vi "Add Tag.vi"() -> ()   [LabVIEW 2017, in "Mustache.lvlib" / "Parser.lvclass"]
uses:
  Parser.lvclass
  Public/Controls/Token Types.ctl
panel:
  out "Parser Out":refnum<class "Parser.lvclass">
  out "Error Out":errorcluster
  in  "Error In":errorcluster
  in  "Parser In":refnum<class "Parser.lvclass">
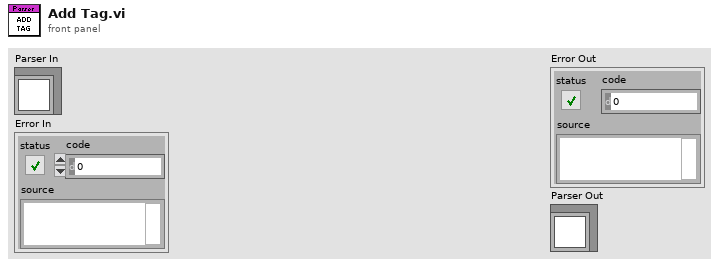
[diagram p1: front panel]
types:
  T1 = typedef "Mustache.lvlib/Parser.lvclass/Token Types.ctl" = enum16{"Text", "Escaped Tag", "Unescaped Tag", "Section", "Incomplete Section", "Partial"}
  T2 = typedef "Mustache.lvlib/Parser.lvclass/Token.ctl" = cluster{"Type":T1, "Data":variant}
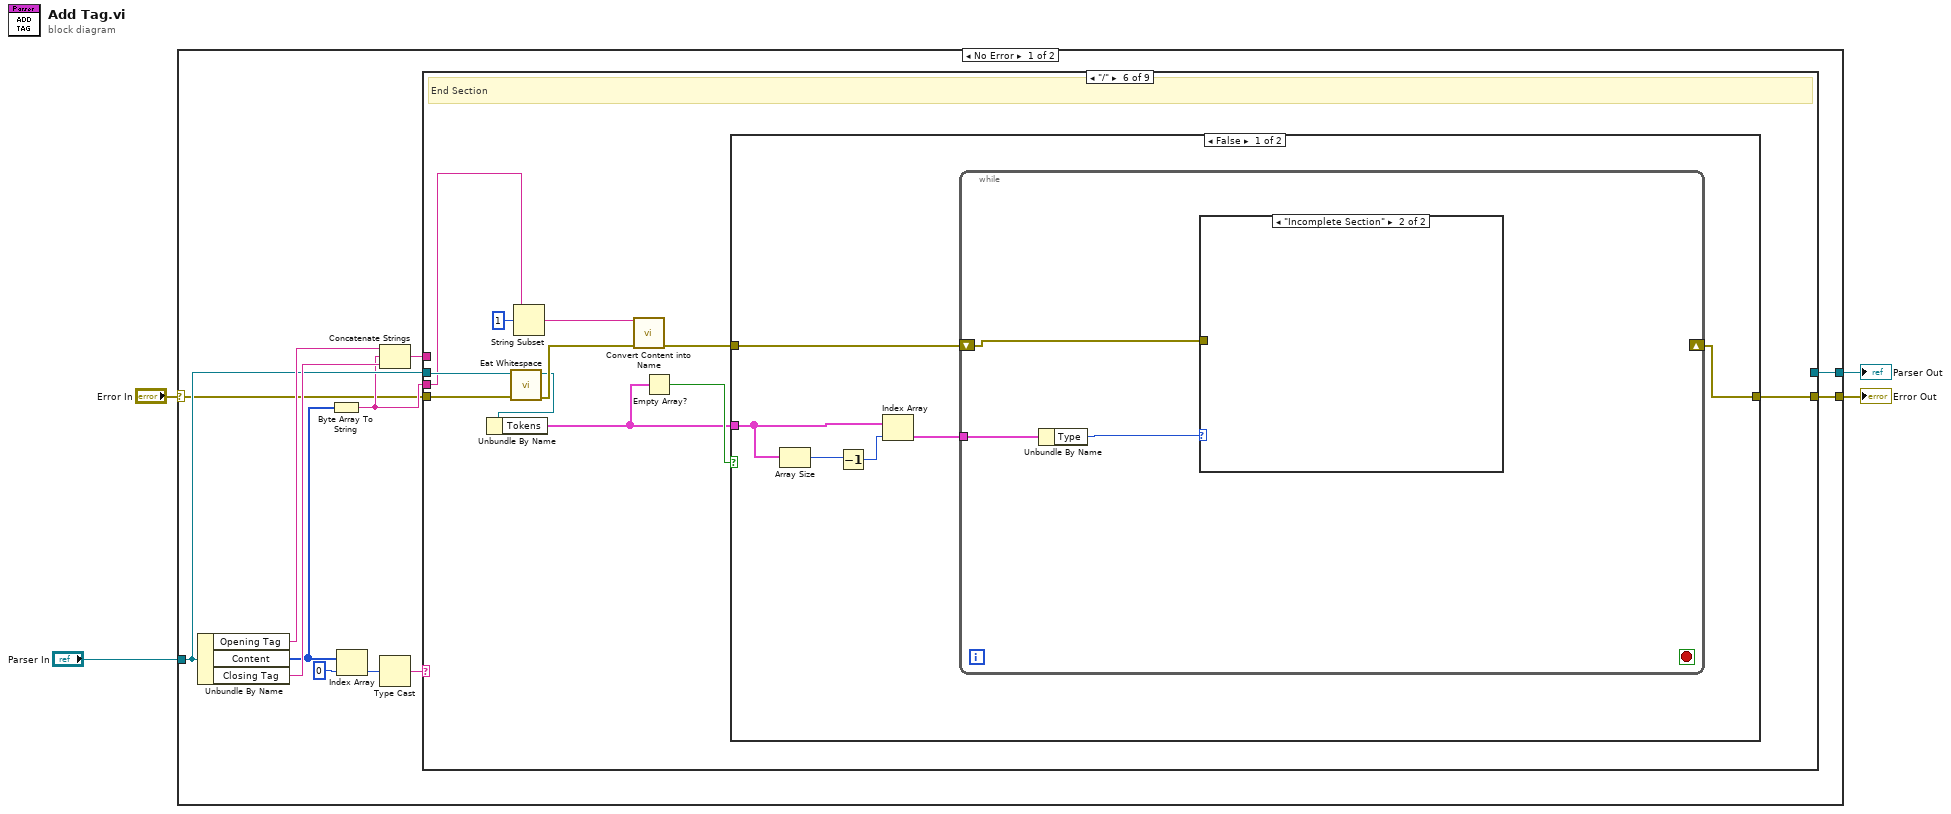
[diagram p0: block diagram]
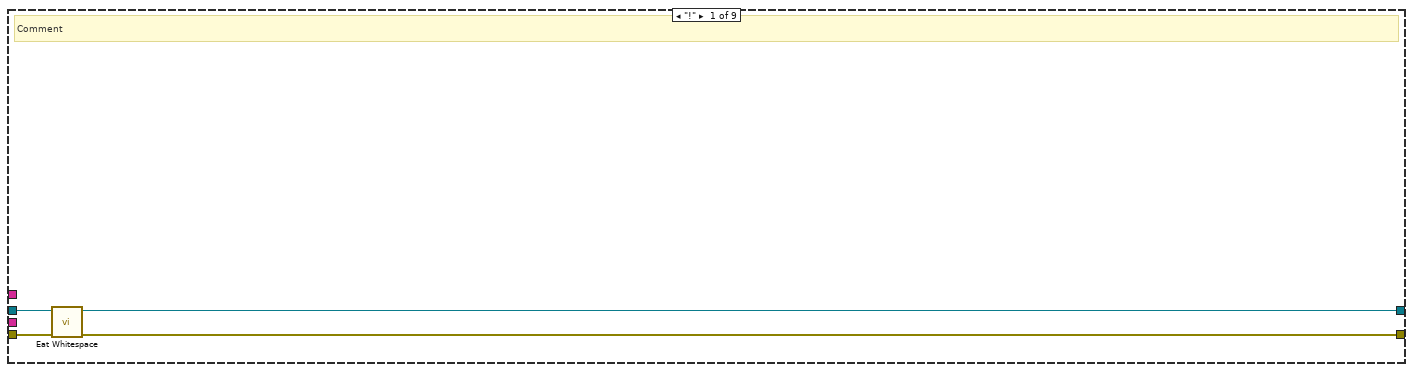
[diagram p2: hidden frame]
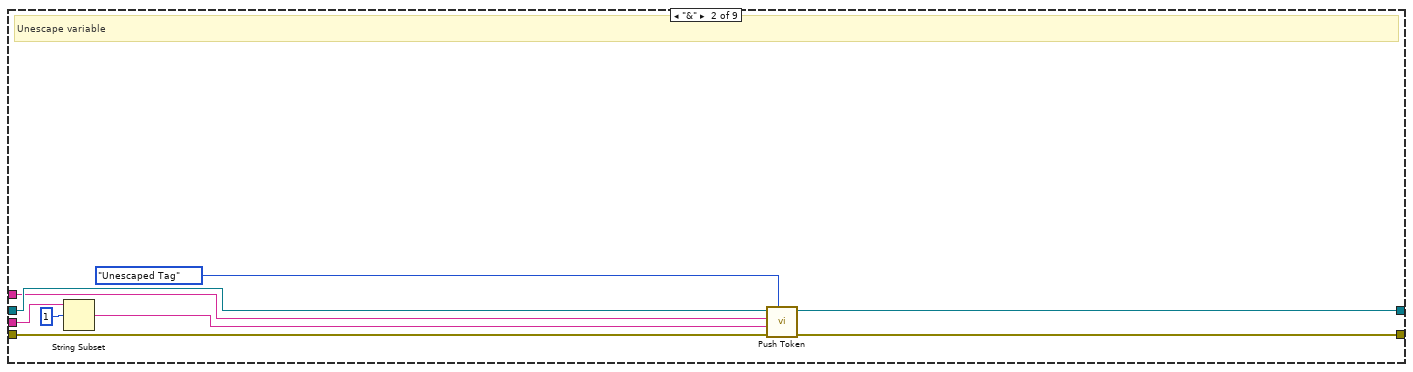
[diagram p3: hidden frame]
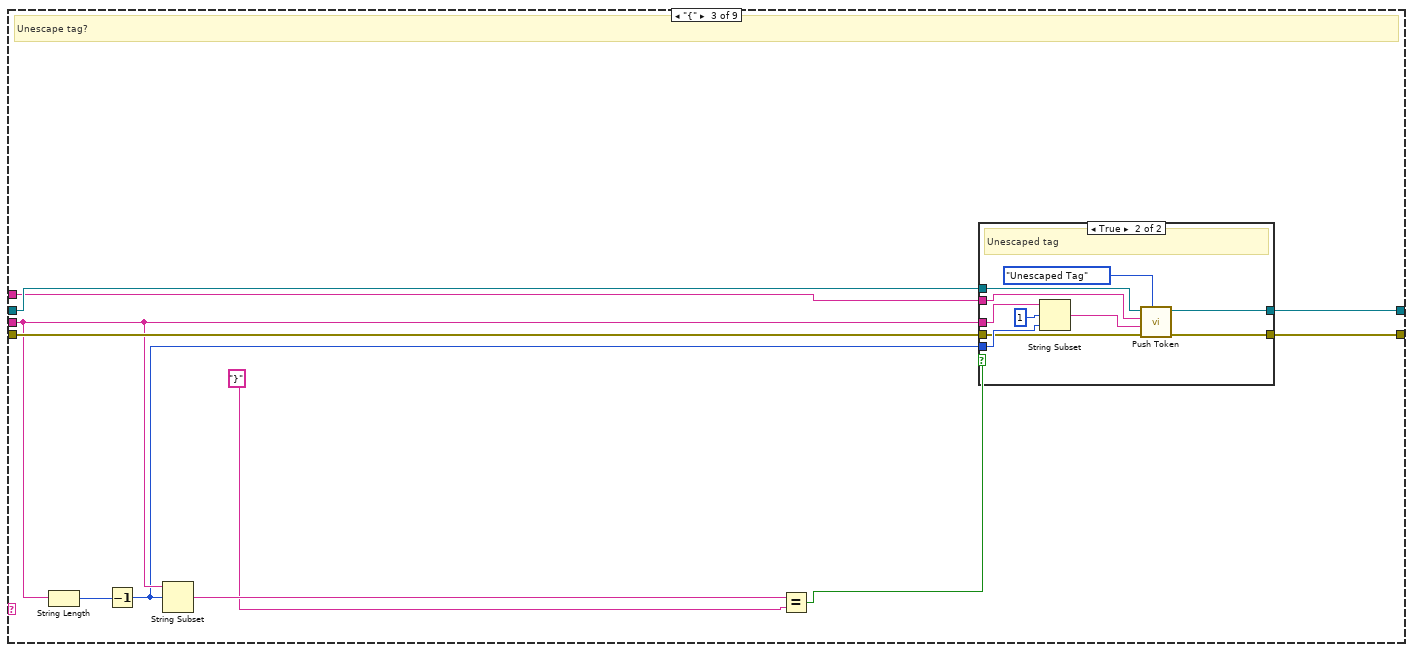
[diagram p4: hidden frame]
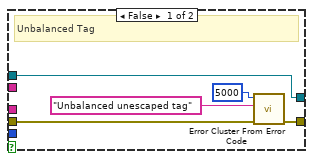
[diagram p5: hidden frame]
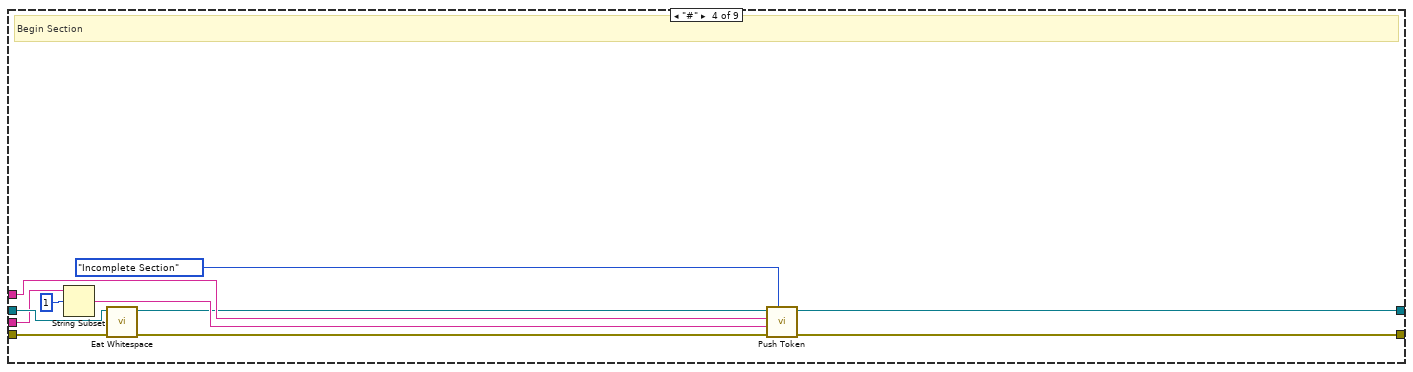
[diagram p6: hidden frame]
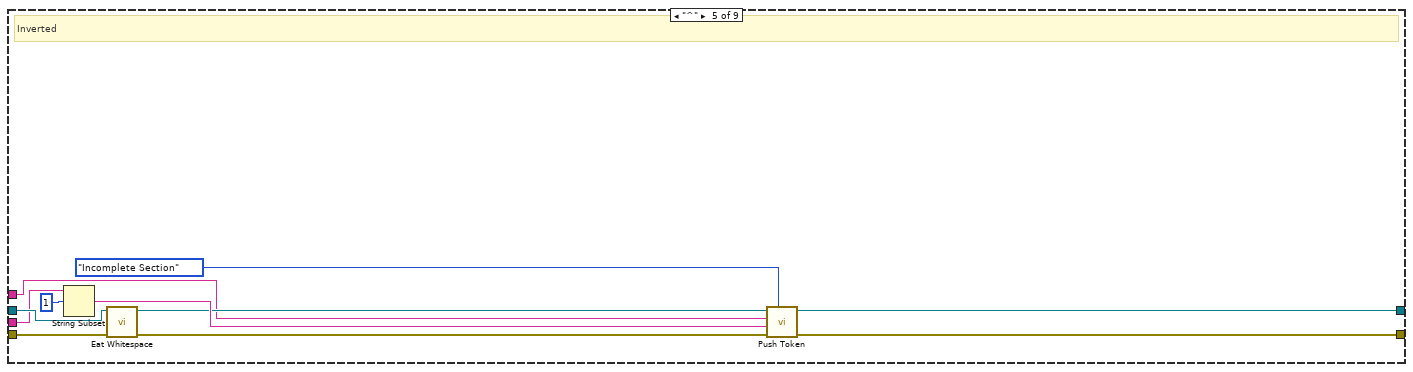
[diagram p7: hidden frame]
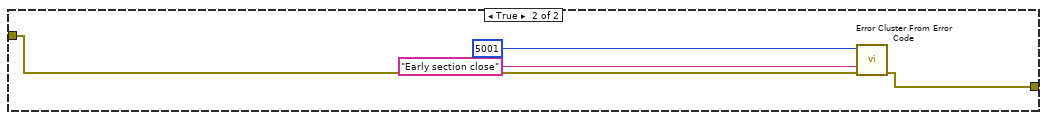
[diagram p9: hidden frame]
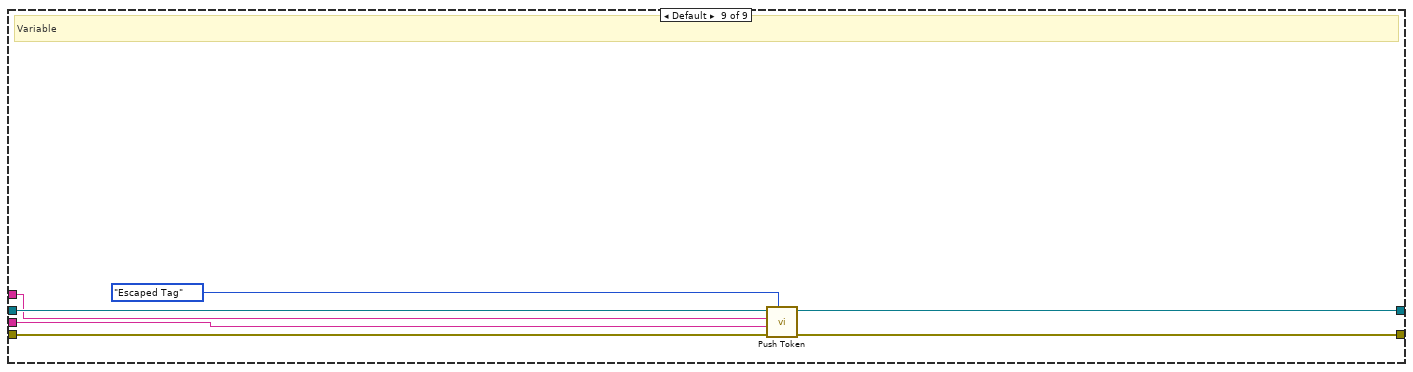
[diagram p12: hidden frame]
diagram:
  n1 = case shown="No Error" "Error In" {
    selector: "Error In" -> [w6 w110]
    tunnel: "Parser In" -> [w10 w109]
    tunnel: [w5 w110] -> w2
    tunnel: [w9 w109] -> w1
    frame No Error {
      n2 = Unbundle By Name(w10) -> ("Opening Tag"=w16:string, "Content"=w14:u8[], "Closing Tag"=w15:string)
      n3 = Byte Array To String(unsigned byte array=w14) -> (string=w7:string)
      n4 = Index Array(array=w14, index=0) -> (element=w12:u8)
      n5 = Concatenate Strings(w16, w7, w15) -> (w8:string)
      n6 = Type Cast(x=w12) -> (*(type *) &x=w11:string)  [unwired: 1 in]
      n7 = case shown="\"/\"" w11 {
        tunnel: w10 -> [w18 w27 w32 w65 w72 w87 _ _ w105]
        tunnel: [w17 w22 w31 w59 w68 _ _ _ w106] -> w9
        tunnel: w8 -> [_ w23 w30 w61 w69 _ _ _ w104]
        tunnel: w7 -> [_ w29 w34 w64 w70 w86 _ _ w103]
        tunnel: w6 -> [w20 w26 w36 w66 w71 w88 _ _ w108]
        tunnel: [w19 w21 w35 w57 w67 w81 _ _ w107] -> w5
        frame "!" {
          # "Comment"
          n8 = call "Eat Whitespace.vi"("Error In"=w20, "Parser In"=w18) -> ("Error Out"=w19:errorcluster, "Parser Out"=w17:refnum<class "Parser.lvclass">)  [unwired: 8 in]
        }
        frame "&" {
          # "Unescape variable"
          n9 = String Subset(string=w29, offset (0)=1) -> (substring=w24:string)  [unwired: 1 in]
          n10 = call "Push Token.vi"("Type"=Token_Types."Unescaped Tag", "Error In"=w26, "Content"=w24, "Tag"=w23, "Parser In"=w27) -> ("Error Out"=w21:errorcluster, "Parser Out"=w22:refnum<class "Parser.lvclass">)  [unwired: 5 in]
        }
        frame "{" {
          # "Unescape tag?"
          n11 = String Length(string=w34) -> (length=w40:i32)
          n12 = Decrement(x=w40) -> (x-1=w33:i32)
          n13 = String Subset(string=w34, offset (0)=w33) -> (substring=w39:string)  [unwired: 1 in]
          n14 = Equal?(x=w39, y="}") -> (x = y?=w37:bool)
          n15 = case shown="True" w37 {
            tunnel: w36 -> [w43 w52]
            tunnel: [w45 w50] -> w35
            tunnel: w34 -> [_ w55]
            tunnel: w33 -> [_ w54]
            tunnel: w32 -> [w41 w51]
            tunnel: [w41 w49] -> w31
            tunnel: w30 -> [_ w47]
            frame False {
              # "Unbalanced Tag"
              n16 = call <vilib>:"Error Cluster From Error Code.vi"("error in (no error)"=w43, "error message (\"\")"="Unbalanced unescaped tag" ("format string"), "error code (0)"=5000) -> ("error out"=w45:errorcluster)  [unwired: 6 in]
            }
            frame True {
              # "Unescaped tag"
              n17 = String Subset(string=w55, offset (0)=1, length (rest)=w54) -> (substring=w46:string)
              n18 = call "Push Token.vi"("Type"=Token_Types."Unescaped Tag", "Error In"=w52, "Content"=w46, "Tag"=w47, "Parser In"=w51) -> ("Error Out"=w50:errorcluster, "Parser Out"=w49:refnum<class "Parser.lvclass">)  [unwired: 5 in]
            }
          }
        }
        frame "#" {
          # "Begin Section"
          n19 = String Subset(string=w64, offset (0)=1) -> (substring=w62:string)  [unwired: 1 in]
          n20 = call "Eat Whitespace.vi"("Error In"=w66, "Parser In"=w65) -> ("Error Out"=w56:errorcluster, "Parser Out"=w60:refnum<class "Parser.lvclass">)  [unwired: 8 in]
          n21 = call "Push Token.vi"("Type"=Token_Types."Incomplete Section", "Error In"=w56, "Content"=w62, "Tag"=w61, "Parser In"=w60) -> ("Error Out"=w57:errorcluster, "Parser Out"=w59:refnum<class "Parser.lvclass">)  [unwired: 5 in]
        }
        frame "^" {
          # "Inverted"
          n22 = String Subset(string=w70, offset (0)=1) -> (substring=w76:string)  [unwired: 1 in]
          n23 = call "Eat Whitespace.vi"("Error In"=w71, "Parser In"=w72) -> ("Error Out"=w73:errorcluster, "Parser Out"=w75:refnum<class "Parser.lvclass">)  [unwired: 8 in]
          n24 = call "Push Token.vi"("Type"=Token_Types."Incomplete Section", "Error In"=w73, "Content"=w76, "Tag"=w69, "Parser In"=w75) -> ("Error Out"=w67:errorcluster, "Parser Out"=w68:refnum<class "Parser.lvclass">)  [unwired: 5 in]
        }
        frame "/" {
          # "End Section"
          n25 = call "Eat Whitespace.vi"("Error In"=w88, "Parser In"=w87) -> ("Error Out"=w83:errorcluster, "Parser Out"=w80:refnum<class "Parser.lvclass">)  [unwired: 8 in]
          n26 = Unbundle By Name(w80) -> ("Tokens"=w78:T2[])
          n27 = String Subset(string=w86, offset (0)=1) -> (substring=w84:string)  [unwired: 1 in]
          n28 = call "Convert Content into Name.vi"("Error In"=w83, "Content"=w84) -> ("Error Out"=w82:errorcluster)  [unwired: 8 in, 1 out]
          n29 = Empty Array?(array=w78) -> (empty?=w79:bool)
          n30 = case shown="False" w79 {
            tunnel: w82 -> [w94 w100]
            tunnel: [w93 w101] -> w81
            tunnel: w78 -> [w92 _]
            frame False {
              n31 = Array Size(array=w92) -> (size(s)=w91:i32)
              n32 = Decrement(x=w91) -> (x-1=w90:i32)
              n33 = Index Array(array=w92, index=w90) -> (element=w89:T2)
              n34 = while {
                shift-right: [_] -> w93
                shift-left: w94 -> [w95]
                tunnel: w89 -> [w97]
                stop <- _ stop-if-true
                n35 = Unbundle By Name(w97) -> ("Type"=w96:T1)
                n36 = case shown="\"Incomplete Section\"" w96 {
                  tunnel: w95 -> [_ _]
                  frame "Text", Default {
                  }
                  frame "Incomplete Section" {
                  }
                }
              }
            }
            frame True {
              n37 = call <vilib>:"Error Cluster From Error Code.vi"("error in (no error)"=w100, "error message (\"\")"="Early section close" ("error message (\"\")"), "error code (0)"=5001) -> ("error out"=w101:errorcluster)  [unwired: 6 in]
            }
          }
        }
        frame ">" {
          # "Partial"
        }
        frame "=" {
          # "Change delimiters"
        }
        frame Default {
          # "Variable"
          n38 = call "Push Token.vi"("Type"=Token_Types."Escaped Tag", "Error In"=w108, "Content"=w103, "Tag"=w104, "Parser In"=w105) -> ("Error Out"=w107:errorcluster, "Parser Out"=w106:refnum<class "Parser.lvclass">)  [unwired: 5 in]
        }
      }
    }
    frame Error {
    }
  }
  "Error Out" <- w2
  "Parser Out" <- w1
